vi "Create Sessions - NSess.vi"(7 "option string":string, 8 "error in":errorcluster, 9 "reset":bool, 11 "session reservation in":refnum<class "Session Reservation.lvclass">) -> (0 "error out":errorcluster, 1 "channel lists":string[](array[string]), 2 "sessions":refnum<k15>[](array[refnum]), 3 "session reservation out":refnum<class "Session Reservation.lvclass">)   [LabVIEW 2020, in "MeasurementLink niDCPower.lvlib"]
doc: "Create the NI-DCPower driver sessions from a reservation."
uses:
  MeasurementLink niDCPower.lvlib
  MeasurementLink Session Management/Session Reservation/Session Reservation.lvclass
  MeasurementLink Session Management/Session Reservation/Session Reservation.lvclass/Session Reservation.ctl
  b3cb301c-7684-4518-818f-a956a366db36.vi
  MeasurementLink Session Management/Session Reservation/Create Sessions Impl.vi
  MeasurementLink Session Management/Session Reservation/Helpers/Get gRPC Device Server Location.vi
  Instrument/Instrument.lvclass
  \\tsclient\C/dev/measurementlink-labview/Source/Runtime/MeasurementLink Instrument/IInstrument/IInstrument.lvclass
  MeasurementLink gRPC Utilities/Service Location FGV.vi
  MeasurementLink Measurement Server/Helpers/Error Strings Global Internal.vi
  <vilib>/Utility/error.llb/Error Cluster From Error Code.vi
  MeasurementLink Instrument/IInstrument/IInstrument.lvclass
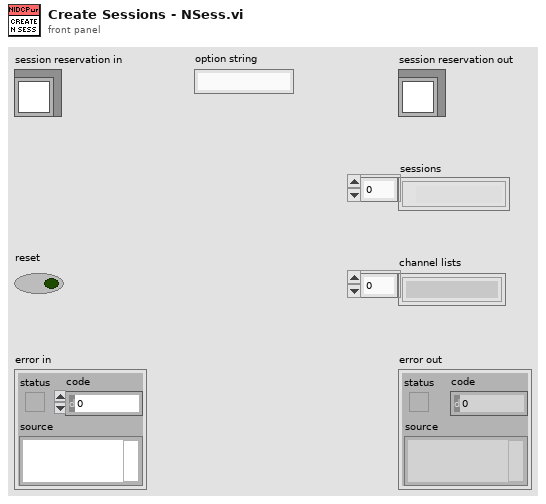
[diagram p1: front panel]
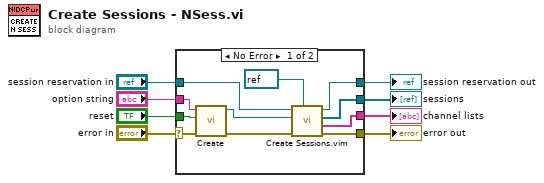
[diagram p0: block diagram]
diagram:
  n1 = case shown="No Error" "error in" {
    selector: "error in" -> [w18 w21]
    tunnel: [w13 w21] -> w7
    tunnel: [w15 w20] -> w5
    tunnel: "session reservation in" -> [w16 w20]
    tunnel: "option string" -> [w19 _]
    tunnel: "reset" -> [w17 _]
    tunnel: [w12 _] -> w2
    tunnel: [w11 _] -> w1
    frame No Error {
      n2 = call "Create.vi"("error in"=w18, "reset"=w17, "option string"=w19) -> ("error out"=w14:errorcluster, "instrument out"=w9:refnum<class "Instrument.lvclass">)  [unwired: 7 in]
      n3 = call "Create Sessions.vim"("session type"=refnum<k15> refnum ("instrument handle out"), "error in"=w14, "instrument in"=w9, "session reservation in"=w16) -> ("error out"=w13:errorcluster, "channel lists"=w11:string[], "sessions"=w12:refnum<k15>[], "session reservation out"=w15:refnum<class "Session Reservation.lvclass">)  [unwired: 4 in]
    }
    frame Error {
    }
  }
  "error out" <- w7
  "session reservation out" <- w5
  "sessions" <- w2
  "channel lists" <- w1
